vi "Read rotAngle.vi"(8 "error in (no error)":errorcluster, 11 "MccRotMove in":refnum<class "MccRotMove.lvclass">) -> (0 "error out":errorcluster, 2 "rotAngle":dbl[unit] min=0.0 max=6.283185307179586, 3 "MccRotMove out":refnum<class "MccRotMove.lvclass">)   [LabVIEW 2022 SP3, in "TCSDataDefinitions.lvlib" / "TCSMountControlCommand.lvlib" / "CommandsForRotatorAxis.lvlib" / "MccRotMove.lvclass"]
uses:
  MccRotMove.lvclass
  MccRotMove.lvclass/MccRotMove.ctl
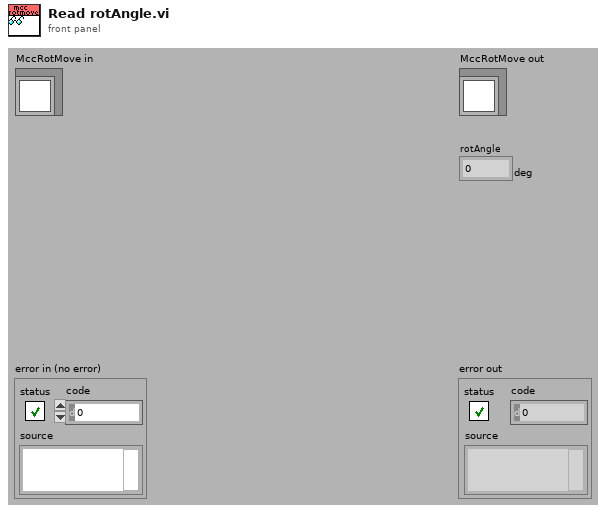
[diagram p1: front panel]
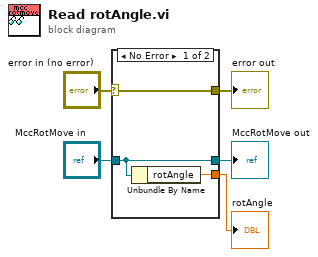
[diagram p0: block diagram]
diagram:
  n1 = case shown="No Error" "error in (no error)" {
    selector: "error in (no error)" -> [w8 w9]
    tunnel: [w8 w9] -> w4
    tunnel: [w7 w10] -> w2
    tunnel: "MccRotMove in" -> [w7 w10]
    tunnel: [w6 _] -> w1
    frame No Error {
      n2 = Unbundle By Name(w7) -> ("rotAngle"=w6:dbl[unit])
    }
    frame Error {
    }
  }
  "error out" <- w4
  "MccRotMove out" <- w2
  "rotAngle" <- w1
